vi "2023_day16_Task2.vi"() -> ()   [LabVIEW 2021]
uses:
  45de9bef-49e1-442e-b527-3241b48d18bf.vi
panel:
  out "Task 2":i32
  in  "Switch":bool caption="Ex. Data  vs.  User Data"
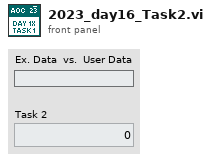
[diagram p1: front panel]
types:
  T1 = cluster{"Map":string[][], "Direction":enum16{"UP", "LEFT", "DOWN", "RIGHT"}, "Position (Row,Col)":i32[], "Energized Tiles":i32[][]}
  T2 = cluster{"Map":string[][], "Direction":enum16{"UP", "LEFT", "DOWN", "RIGHT"}, "Position (Row,Col)":i32[], "Energized Tiles":i32[][]}[][]
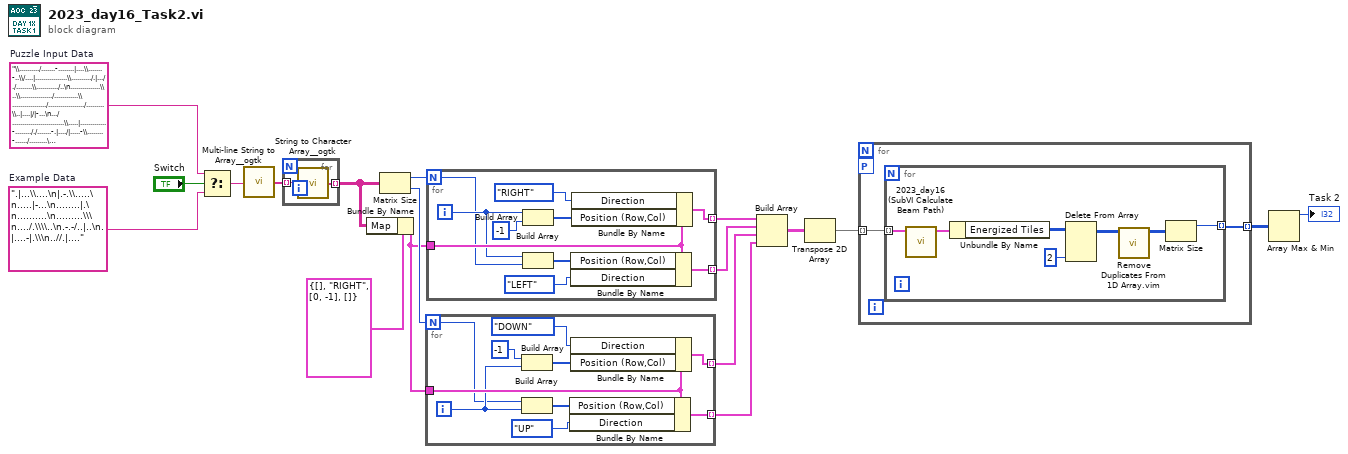
[diagram p0: block diagram]
diagram:
  w16 = "\\........../.......-........|....\\.......-..\\/....|................\\........../.|..././........\\.........../..\n...............\\..\\................/............\\................./................../.........\\..|....|/|-...\n.../..........................\\.....|.............-.......././.......-.|..../|.....-\\........-....../.........\n|..........................-..........-......./............................-..|................-..............\n.....|......../...../.......-.\\..............................-........|............|/.../../........./........\n..\\...|..-......\\.........-\\.||........|./................\\....\\........-..\\..................../..\\....-...|.\n.|...........|............-........./.-.................|.|....../...............|..../..-..-...\\...........|.\n..............\\............................................................./......................./\\....-...\n./........|...\\.\\..|..-....\\............................|........./.................|/...............-........\n\\....\\./.............../................../....|......./........../.\\......./........-....\\......../....../|..\n./......--..........\\..|.--........-...../......./........\\.....|/..................|//...........|.........-.\n.......|.....\\-.\\..-......-.........|.....................-/\\.....-..........|.............-....\\.....\\.-.....\n..--...\\....-..|..................................-......-......\\......-................\\...../..-/....--.....\n....-.........................\\.\\............|...............|.....-...\\....|-................................\n.................-..|.\\..\\....-..........|...../.....-...-.-../.............../................-..............\n-..-......|..............................\\.....\\........|...../........\\.................../..................\n..............-.....-.|..........|.\\..................|........|...........\\.\\...|........-...................\n..\\............/...\\\\........../...-..\\.../.........\\..|................../......\\..-.../....................\\\n..................|...\\......................./...|......../..............-./...\\........\\......./|...\\..-..-.\n.................................................-................|.........................................\\.\n......-...............................|./............./...........................-\\/..../......\\..........\\..\n......\\....|..........................\\.-|..........................|....................\\.....\\/...-.........\n..\\..-|...|.....-...../......./....|...............\\................|..|.......\\...........................-..\n..\\......-.......\\.........\\................|...........|....../...../..........-./...-|..................../.\n................./.......\\...|.....\\....-................./......../..\\...........-...|.../|................\\.\n..|..\\./.........\\.\\.......................-......|....-..../.../................-.......\\../.../...../.......\n........../........./..|..-....................\\\\............\\........................-......-......|.........\n.../-....\\..\\..........\\....\\\\......................................./........\\...-.................\\.........\n................................../.................|..\\.-..|................|/....-.........................|\n...-.................||..../....................-..........................................|.-................\n..//.\\..........................|.....|-.............\\.\\......-....\\.\\.......\\............-..............\\-...\n.......|.|..-........./..|........-.....|........................-...................-......\\................-\n..-..|..........|....-.............|.|/...../../..................\\...\\................../......|....|........\n........\\..././.............../.............../....-../.....|....\\................|/.../.....|.|-..|..........\n......|..........\\...-./........-...............................\\..........|.............|..\\..|......./.....|\n.............................-................................................|................/......\\.../..-\n......-........\\..........-..../...............\\............/.....\\......|........................-.|.../.....\n...\\...............-....-........-............-...../....|.\\.../.......\\..-....................|........|.....\n.............................-...\\....|...|.......\\............................-............\\.................\n....................|...-........-.........-..\\................/....................../.|.......-.............\n......\\.........................../....-....|...........................................\\...-.........|......\\\n.............\\../\\..............|\\.\\..........|\\.../..................../\\...................|\\.......\\.......\n/.................../.\\\\.........................../...........-...-..........-..-............................\n............\\......../........-.........../........./.................-................./...........|.........\n.........\\.......|.......\\........./.....................\\..............\\\\....../...|-....\\..|..-.....|.......\n.|....-.............\\.........\\.\\../.......-...........................\\./..........................--\\......\\\n........./..../................./.................\\............................................./../.\\........\n.....-..............-.-...\\/..|....-........./.....................\\................./.\\..........-...|....|..\n........|...|.-.......|.......-............\\.../....|...\\............../............-.........................\n........................|.....\\........................./\\/.........................|.........................\n....\\..././..........|.....\\......................-................./.....|...............................|-..\n.../.........../.-......\\..../.................-...\\.....-......\\.....\\..............//.|..............-..-...\n....../............./-/.\\...........\\...\\..|/........................-...../......\\........-./\\..........||...\n.................................../............|....................../..|.....\\......\\............/.........\n.....|....\\...|.-./............................./..-....|.\\.......................-../.-..-.........\\.........\n..........\\...|../.......-|............-........../...../..........-......-../.-......|..../.-.../............\n.-.........-............|/.......-........|...................-.........-........../.-........\\..........|/...\n.........\\.........\\....../....|...\\\\......-..........-................\\................................-.....\n............-...../......|...//........\\-....|......../........./..................-................../....--.\n...............|.................................|.../...\\....................\\................|...\\.|........\n..............\\.........\\.........\\....|.-.......\\.\\........-.........../...|.....|..............\\.......\\....\n........-.-.....|.../......-\\..|.....-.........|.-................\\......./....\\...-.....\\..|/...............|\n....|.....................-...................\\......\\......-.......................-...../........./....\\....\n..|...|.......\\./..-..............\\.............................................\\../....|.....................\n..................-../........|.....-\\.../................................................./..\\...|......-...-\n.....\\......\\........\\.....................|...|../......../....../.\\........./...............................\n............../........../...........\\..\\/..|.\\...|..........-................................\\-..............\n/...............\\...|......\\............/|...................|....././...\\............................-.|.....\n...........|................/-......\\.....-.........-.............../......./............../|.................\n..-...........|..\\.............\\....|/...............|..../..............\\...............|./......|........./.\n.....\\\\..|......\\....\\.......-.................\\.-......................|........./...|.........|...|...-.....\n-...../....|....../............./.......|/../\\.............../...../-\\.../-.......|........../..............\\\\\n..........\\....................../.................|...--../..................................................\n.\\.................../......|......-.............................//......|.../|.|....\\.............\\..........\n.\\-...........-.........|..................................../........|......../...-............\\....-...-....\n......\\......|................-...../....|........-..\\.....-........//................../.....|.........-.....\n.....-..........-.|/.........-....................../......|.|./........................................./\\\\|.\n...\\................|.........../..-....|..-..........|........../....-....../......./.....-..\\.....\\\\..../...\n.....\\.....-..................-...-..../....|....|.................|...\\./.............../.......|.\\/...../...\n.||......../........../.-...|...........\\.................\\........-........|........................-...|....\n........./......\\......|...............\\.\\.................................................\\.................|\n..........................|....................|..../-...............|....|......../....-..................|..\n.-........\\.|......../...|...................|.........|............\\.....|.......\\........./.................\n................-........................\\...........|................../................-.............\\......\n.......\\..........|.............../...|.-......................../....\\.............-.......\\./...............\n..........\\...........................................-........|.......\\........./...-........\\...............\n../......./...\\|...............-........\\................./...\\...................../.....-.-....-...........-\n.\\../......../....-\\................................|.....-..|...............................-................\n..........................\\.....|................/.....\\......../.............|..............\\......./-..|....\n|.........-.|............./......-.................|.......|...\\/...........|...........................\\\\....\n-..................|.........................-.............-.....|..../.........\\...-/.....|............/\\....\n.........\\.\\....\\...........|....-.../..............|.....|-.......\\.............-......./......././.......\\..\n..../.....-...........................................\\.../..\\.|.......................-..//....-......|......\n./-..................\\..\\....................................\\......./.\\....|.................................\n...../....................................-....-/........................-/.........-.\\...|......./..-.\\......\n.....|.............-.......|-..-.................................|-...........................\\.|.....|.......\n.........\\-.............\\.............../....-....|....-.|..........\\............|.\\...|.....-................\n............/.......-....|./....|../..../......./..\\.................-..................|.....................\n../....-........./.....\\...............\\......-....|...\\........../.....|........................\\............\n...../.\\.............\\.........................-..|.......|......-......|................./......./-..........\n...\\..........\\.......................\\.-..././.........|..\\..................\\...../...|.......|............-\n........./............-..................................|.....................-..............................\n........................|.....\\.........\\..............-..\\..........||...../.\\\\./....../.....................\n.................-.............\\.../...........\\...\\......--................\\.....\\.............\\....-........\n.../-..........\\.\\............-.......-.............\\..\\.\\...../........|...-..-..|..........\\................\n\\.|..\\......\\-......./.........||..\\.........................................................-...../..........\n....|..........................................\\......-..........\\.../...\\-........|..........................\n.......-.......\\..//./....|...............\\.\\..-...\\....|....................-......\\......\\..-......../......\n/..../../....-../....-....-......................\\........./..........-/..\\......./..\\-.../..........|........\n.|....\\\\........./....\\.............-......--\\...........|.........|..\\...................../........./.\\....."  # Puzzle Input Data
  w17 = ".|...\\....\n|.-.\\.....\n.....|-...\n........|.\n..........\n.........\\\n..../.\\\\..\n.-.-/..|..\n.|....-|.\\\n..//.|...."  # Example Data
  n1 = Select(t=w16, s="Switch", f=w17) -> (s? t:f=w15:string)
  n2 = call <userlib>:"Multi-line String to Array__ogtk.vi"("string"=w15) -> ("lines"=w14:string[])
  n3 = for {
    tunnel: w14 -> [w20] mode=indexing
    tunnel: [w19] -> w4 mode=indexing
    n4 = call <userlib>:"String to Character Array__ogtk.vi"("Input String"=w20) -> ("Character Array"=w19:string[])
  }
  n5 = Bundle By Name(cluster=T1 {"Map"=[], "Direction"=enum."RIGHT", "Position (Row,Col)"=[0, -1], "Energized Tiles"=[]} ("Beam"), "Map"=w4) -> (w3:T1)
  n6 = Matrix Size(0:w4) -> (1:w12:i32, 2:w8:i32)
  n7 = for {
    N: w8 -> [w24]
    tunnel: w3 -> [w30]
    tunnel: [w23] -> w7 mode=indexing
    tunnel: [w22] -> w6 mode=indexing
    i -> [w25]
    n8 = Build Array(-1, w25) -> (w28:i32[])
    n9 = Build Array(w24, w25) -> (w26:i32[])
    n10 = Bundle By Name(cluster=w30, "Position (Row,Col)"=w26, "Direction"=enum16{"UP", "LEFT", "DOWN", "RIGHT"}."UP") -> (w22:T1)
    n11 = Bundle By Name(cluster=w30, "Direction"=enum16{"UP", "LEFT", "DOWN", "RIGHT"}."DOWN", "Position (Row,Col)"=w28) -> (w23:T1)
  }
  n12 = for {
    N: w12 -> [w34]
    tunnel: w3 -> [w40]
    tunnel: [w33] -> w11 mode=indexing
    tunnel: [w32] -> w10 mode=indexing
    i -> [w35]
    n13 = Build Array(w35, -1) -> (w38:i32[])
    n14 = Build Array(w35, w34) -> (w36:i32[])
    n15 = Bundle By Name(cluster=w40, "Position (Row,Col)"=w36, "Direction"=enum16{"UP", "LEFT", "DOWN", "RIGHT"}."LEFT") -> (w32:T1)
    n16 = Bundle By Name(cluster=w40, "Direction"=enum16{"UP", "LEFT", "DOWN", "RIGHT"}."RIGHT", "Position (Row,Col)"=w38) -> (w33:T1)
  }
  n17 = Build Array(w11, w10, w7, w6) -> (w9:T2)
  n18 = Transpose 2D Array(2D array=w9) -> (transposed array=w2:T2)
  n19 = for {
    tunnel: w2 -> [w42] mode=indexing
    tunnel: [w41] -> w1 mode=indexing
    workers-P: _ -> [_]
    n20 = for {
      tunnel: w42 -> [w44] mode=indexing
      tunnel: [w43] -> w41 mode=indexing
      n21 = call "2023_day16 (SubVI Calculate Beam Path).vi"("Beam in"=w44) -> ("Beam out"=w49:T1)  [unwired: 10 in]
      n22 = Unbundle By Name(w49) -> ("Energized Tiles"=w45:i32[][])
      n23 = Delete From Array(array=w45, index (col)=2 ("disabled index (col)")) -> (array with subset deleted=w47:i32[][])  [unwired: 2 in, 1 out]
      n24 = call "Remove Duplicates From 1D Array.vim"("array"=w47) -> ("array with duplicates removed"=w48:i32[][])  [unwired: 10 in]
      n25 = Matrix Size(0:w48) -> (1:w43:i32)  [unwired: 1 out]
    }
  }
  n26 = Array Max & Min(array=w1) -> (max value=→"Task 2":i32)  [unwired: 3 out]
